vi "Kateter.vi"() -> ()   [LabVIEW 2024]
panel:
  out "Array":dbl[](array[numeric])
  out "Waveform Chart":dynamicdata(graph)
  in  "stop":bool
  out "return value":cluster{dbl, dbl}
  out "error out":errorcluster
  out "appended path":path
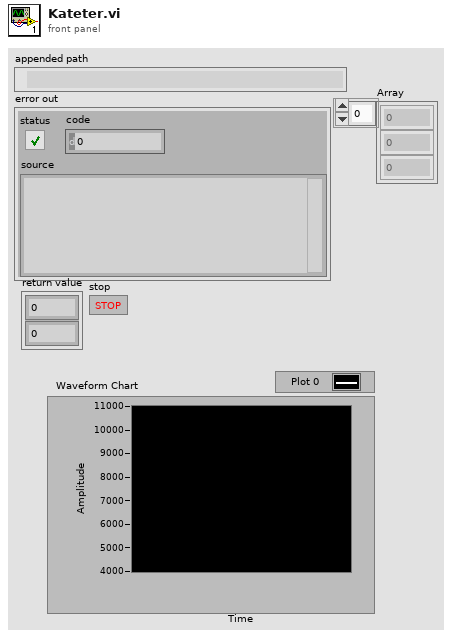
[diagram p1: front panel]
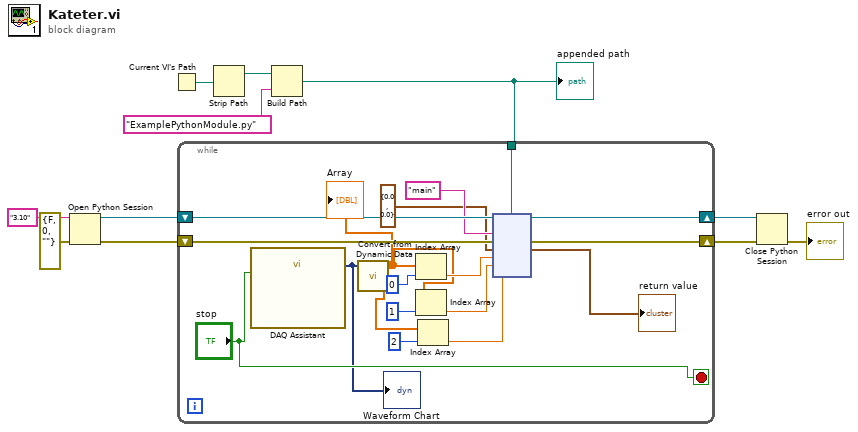
[diagram p0: block diagram]
diagram:
  n1 = Open Python Session(python version="3.10" ("Python version"), 3:errorcluster {"status"=FALSE, "code"=0, "source"=""} ("error in (no error)")) -> (session out=w11:refnum<k35>, error out=w8:errorcluster)  [unwired: 1 in]
  n2 = Current VI's Path() -> (path=w6:path)
  n3 = Strip Path(path=w6) -> (stripped path=w5:path)  [unwired: 1 out]
  n4 = Build Path(base path=w5, name or relative path="ExamplePythonModule.py") -> (appended path=w3:path)
  "appended path" <- w3
  n5 = while {
    tunnel: w3 -> [w24]
    shift-right: [w27] -> w10
    shift-left: w11 -> [w28]
    shift-right: [w26] -> w9
    shift-left: w8 -> [w25]
    stop <- "stop" stop-if-true
    n6 = call "DAQ Assistant"("stop (T)"="stop") -> ("data"=w15:dynamicdata)  [unwired: 16 in, 2 out]
    "Waveform Chart" <- w15
    n7 = call "Convert from Dynamic Data"("Dynamic Data Type"=w15) -> ("Array"=w13:dbl[])  [unwired: 3 in]
    "Array" <- w13
    n8 = Index Array(array=w13, index=0) -> (element=w20:dbl)
    n9 = Index Array(array=w13, index=1) -> (element=w19:dbl)
    n10 = Index Array(array=w13, index=2) -> (element=w12:dbl)
    n11 = node(w28, w24, "main" ("function name"), w25, cluster{dbl, dbl} {0.0, 0.0}, w20, w19, w12) -> (w27:refnum<k35>, w26:errorcluster, →"return value":cluster{dbl, dbl})  [unwired: 3 in, 2 out]
  }
  n12 = Close Python Session(session in=w10, error in=w9) -> (11:→"error out":errorcluster)
